vi "Build Octree from triangles.vi"(3 "Triangle array":T4[](array[typedef]), 4 "World Pmin (x, y, z)":sgl[](array[numeric]), 5 "World Pmax (x, y, z)":sgl[](array[numeric]), 6 "Octree resolution (model units)":sgl) -> (0 "Stack error":errorcluster, 1 "Branch levels":i32, 2 "Octree node array":T1[](array[typedef]))   [LabVIEW 2016]
uses:
  Typedefs/Triangle.ctl
  Typedefs/TreeNodeBox.ctl
  Typedefs/Quad.ctl
  Typedefs/Quadplane enum.ctl
  Subroutines/TriVert-in-Box test.vi
  Subroutines/BoxEdges-Tri intersection test.vi
  Subroutines/TriEdges-Box intersection test.vi
  Subroutines/Point-in-Box test (axis-aligned).vi
  Subroutines/Edge-Tri intersection test.vi
  Subroutines/Edge-Quad intersection test.vi
  Subroutines/Point-in-Tri test.vi
  Subroutines/Edge-Plane intersection test.vi
  Subroutines/Point-in-Quad test (axis-aligned).vi
  Subroutines/Dot product.vi
panel:
  out "Octree node stack history":i32(graph)
  # "PN 17/01/2015"
  # "Vertices"
  # "Edges"
  # "Unit normal"
  # "Plane ident."
  # "Vertices"
  # "Edges"
  # "Unit normal"
  # "Plane ident."
  # "Vertices"
  # "Edges"
  # "Unit normal"
  # "Plane ident."
  # "Vertices"
  # "Edges"
  # "Unit normal"
  # "Plane ident."
  # "Vertices"
  # "Edges"
  # "Unit normal"
  # "Plane ident."
  # "Vertices"
  # "Edges"
  # "Unit normal"
  # "Plane ident."
  # "Vertices"
  # "Edges"
  # "Unit normal"
  # "Edge unit normals"
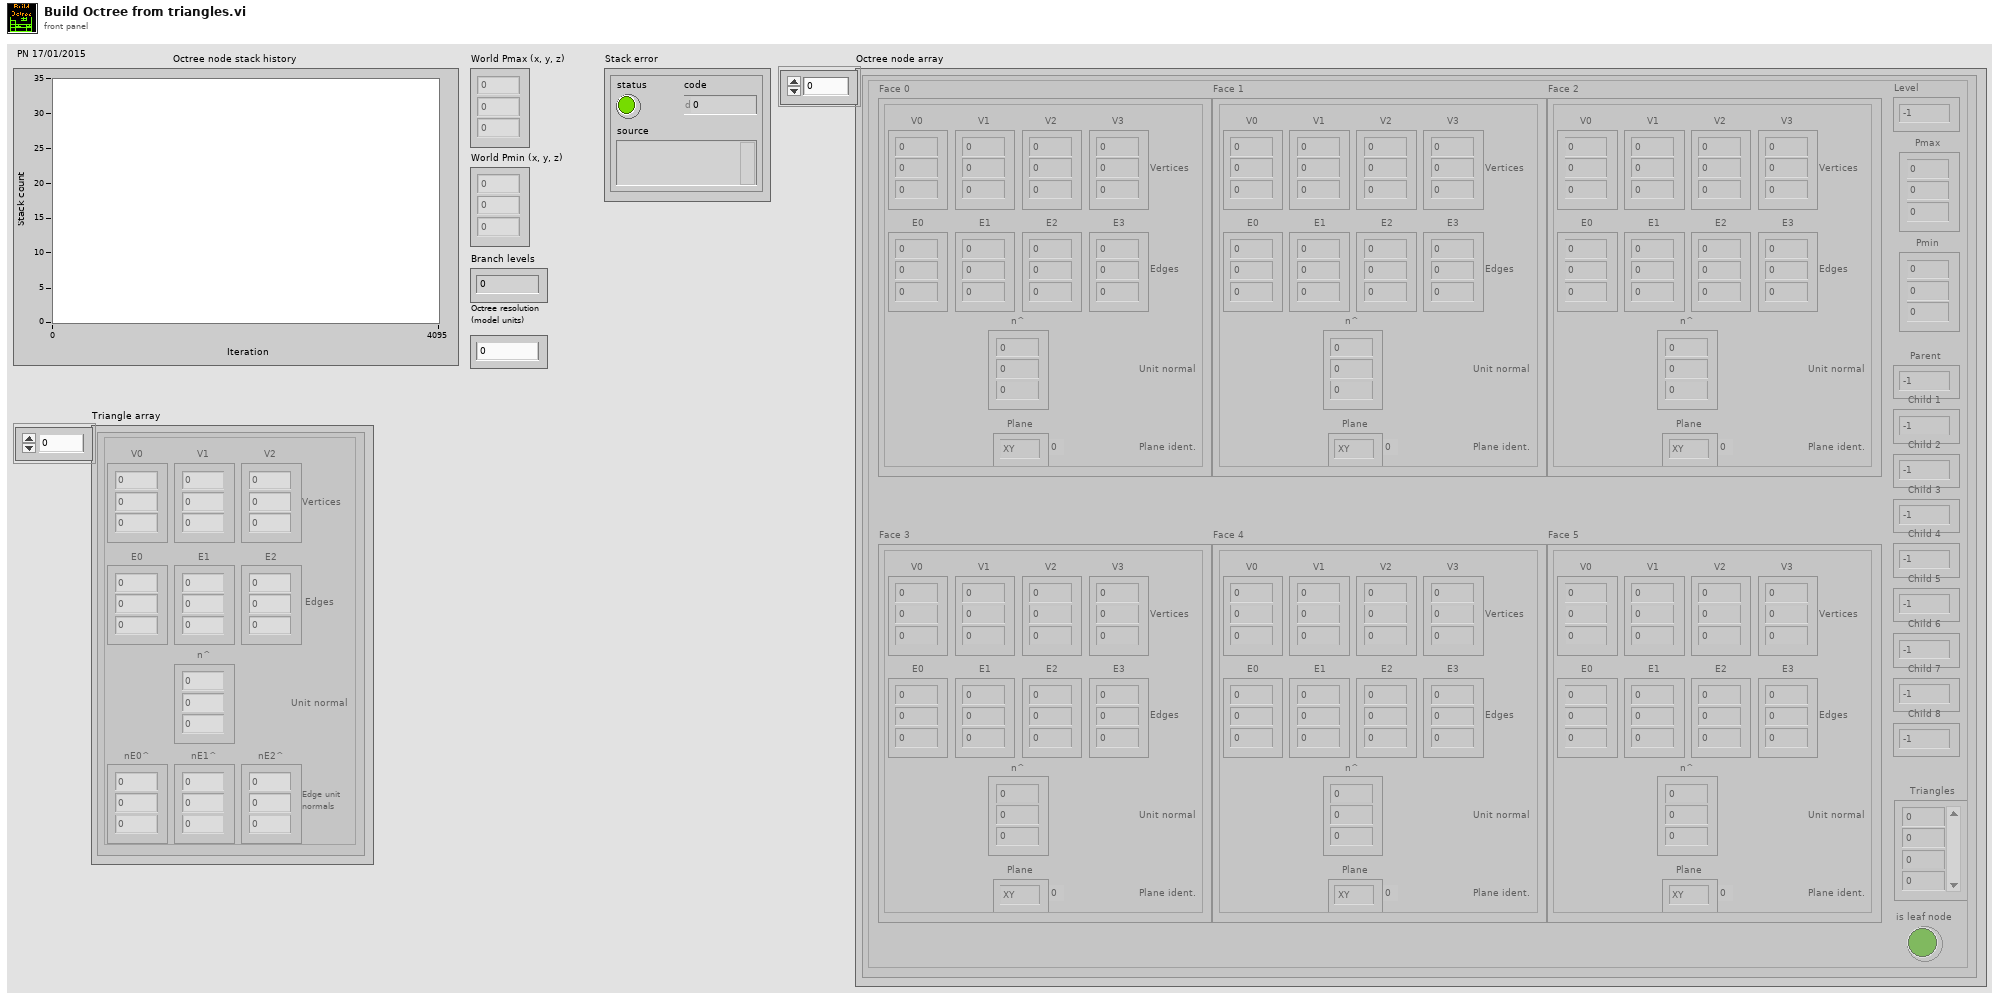
[diagram p1: front panel]
types:
  T1 = typedef "TreeNodeBox.ctl" = cluster{"Face 0":T2, "Face 1":T2, "Face 2":T2, "Face 3":T2, "Face 4":T2, "Face 5":T2, "Level":i32, "Pmax":sgl[], "Pmin":sgl[], "Parent":i32, "Child 1":i32, "Child 2":i32, "Child 3":i32, "Child 4":i32, "Child 5":i32, "Child 6":i32, "Child 7":i32, "Child 8":i32, "Triangles":i32[], "is leaf node":bool}
  T2 = typedef "Quad.ctl" = cluster{"V0":sgl[], "V1":sgl[], "V2":sgl[], "V3":sgl[], "E0":sgl[], "E1":sgl[], "E2":sgl[], "E3":sgl[], "n^":sgl[], "Plane":T3}
  T3 = typedef "Quadplane enum.ctl" = enum8{"XY", "XZ", "YZ", "-XY", "-XZ", "-YZ"}
  T4 = typedef "Triangle.ctl" = cluster{"V0":sgl[], "V1":sgl[], "V2":sgl[], "E0":sgl[], "E1":sgl[], "E2":sgl[], "n^":sgl[], "nE0^":sgl[], "nE1^":sgl[], "nE2^":sgl[]}
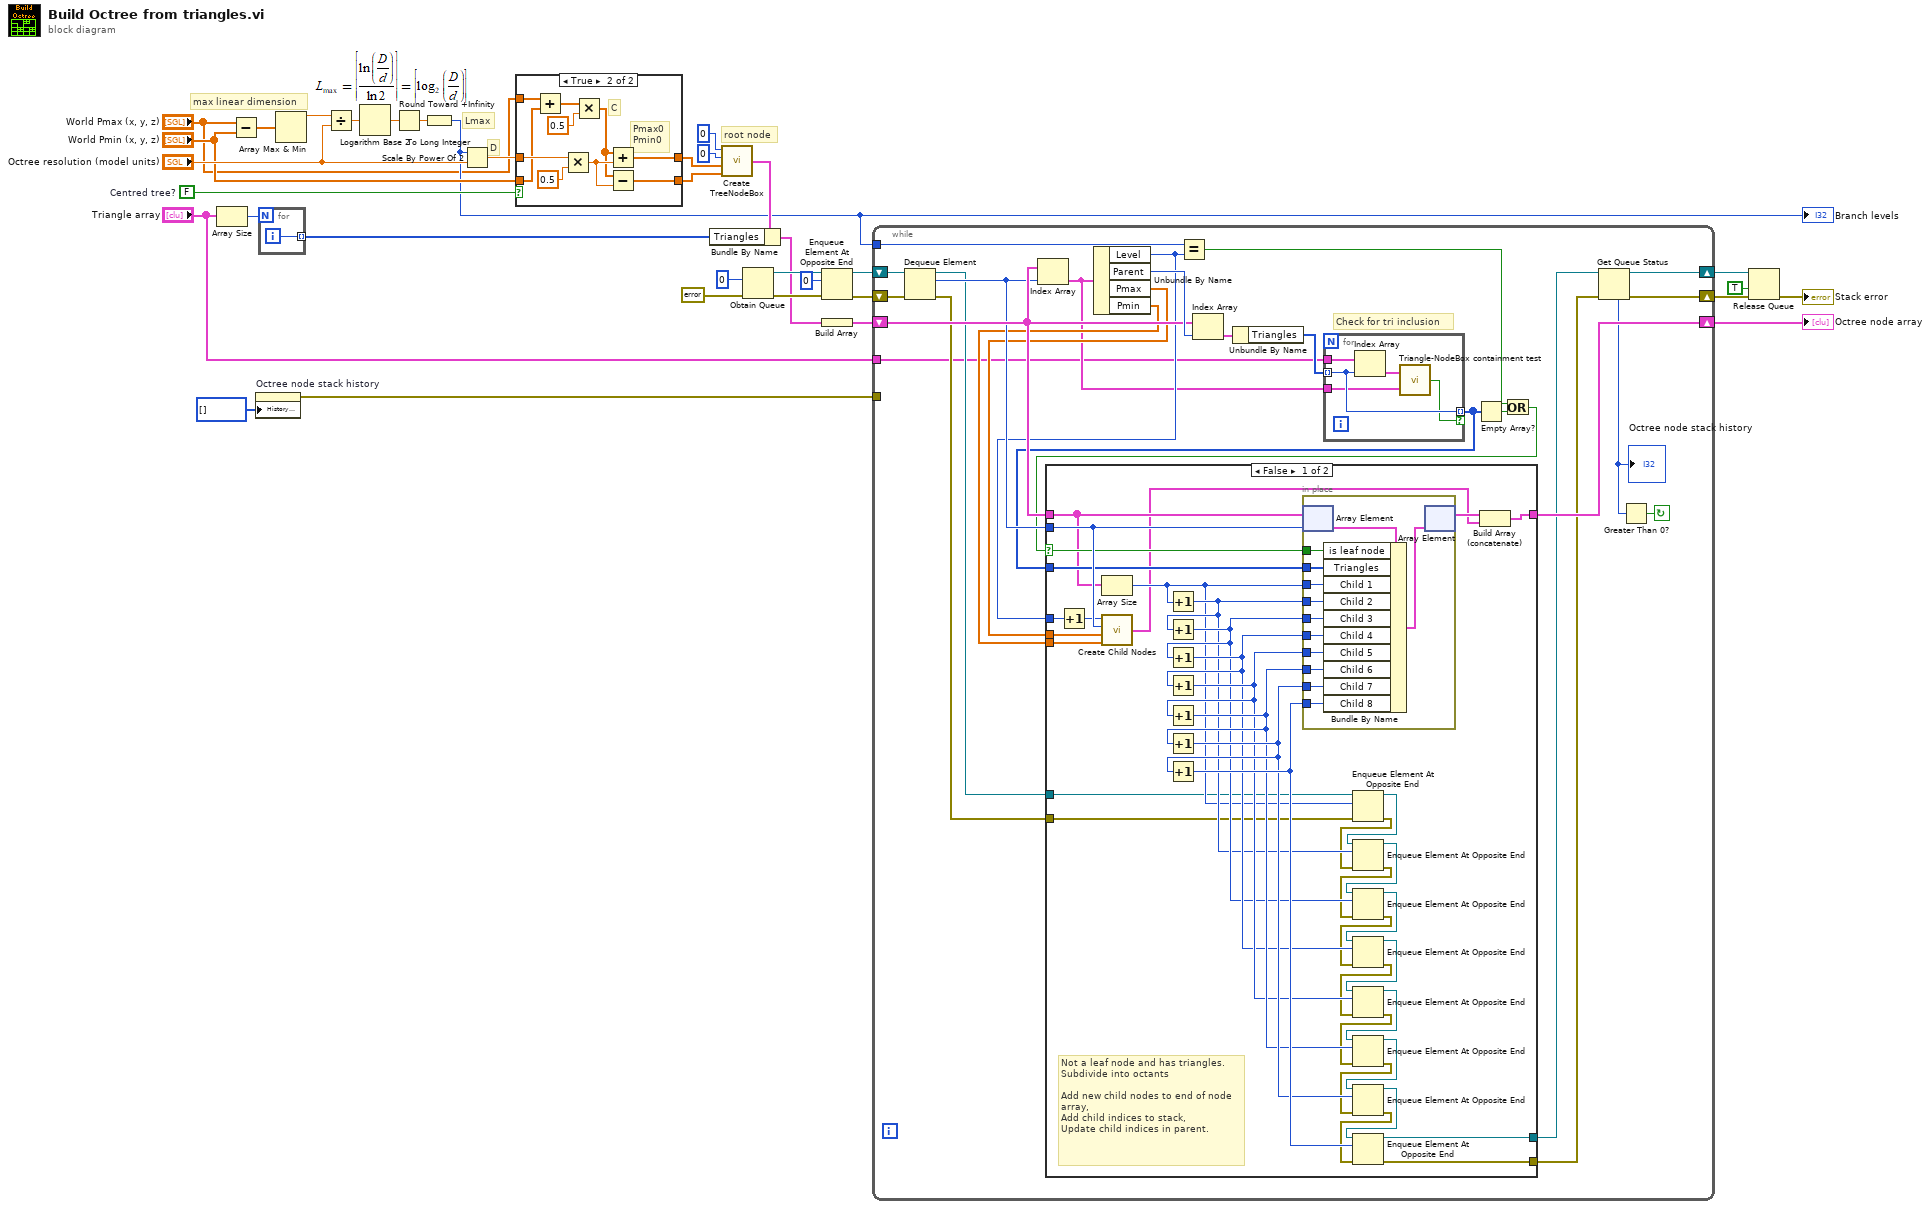
[diagram p0: block diagram]
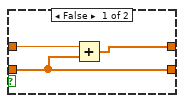
[diagram p2: hidden frame]
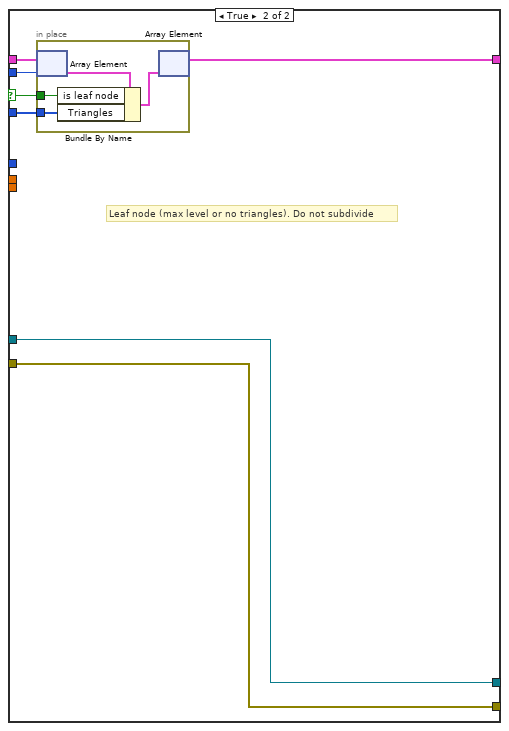
[diagram p3: hidden frame]
diagram:
  w4 = FALSE  # Centred tree?
  # "root node"
  # "D"
  # "Lmax"
  # "max linear dimension"
  n1 = Array Size(array="Triangle array") -> (size(s)=w24:i32)
  n2 = Subtract(x="World Pmax (x, y, z)", y="World Pmin (x, y, z)") -> (x-y=w35:sgl[])
  n3 = property on="Octree node stack history" class="WFChart (strict)"("History Data"=i32[] []) -> (error out=w12:errorcluster)  [unwired: 2 in, 1 out]
  n4 = for {
    N: w24 -> [_]
    tunnel: [w36] -> w23 mode=indexing
    i -> [w36]
  }
  n5 = Array Max & Min(array=w35) -> (max value=w9:sgl)  [unwired: 3 out]
  n6 = Divide(x=w9, y="Octree resolution (model units)") -> (x/y=w34:sgl)
  n7 = Logarithm Base 2(1:w34) -> (0:w33:sgl)
  n8 = Round Toward +Infinity(x=w33) -> (ceil(x): smallest int >= x=w32:sgl)
  n9 = To Long Integer(number=w32) -> (32bit integer=w3:i32)
  "Branch levels" <- w3
  n10 = Scale By Power Of 2(n=w3, x="Octree resolution (model units)") -> (x*2^n=w8:sgl)
  n11 = case shown="True" w4 {
    tunnel: w8 -> [w39 w47]
    tunnel: [w37 w46] -> w5
    tunnel: [w38 w45] -> w6
    tunnel: "World Pmin (x, y, z)" -> [w38 w41]
    tunnel: "World Pmax (x, y, z)" -> [_ w40]
    frame False {
      n12 = Add(x=w39, y=w38) -> (x+y=w37:sgl[])
    }
    frame True {
      # "C"
      # "Pmax0\nPmin0"
      n13 = Add(x=w40, y=w41) -> (x+y=w44:sgl[])
      n14 = Multiply(x=w47, y=sgl 0.5 ("Numeric")) -> (x*y=w48:sgl)
      n15 = Multiply(x=w44, y=sgl 0.5 ("Numeric")) -> (x*y=w42:sgl[])
      n16 = Add(x=w42, y=w48) -> (x+y=w46:sgl[])
      n17 = Subtract(x=w42, y=w48) -> (x-y=w45:sgl[])
    }
  }
  n18 = call "Create TreeNodeBox.vi"("Pmin"=w6, "Pmax"=w5, "Parent"=0, "Level"=0) -> ("Box"=w15:T1)
  n19 = Bundle By Name(cluster=w15, "Triangles"=w23) -> (w22:T1)
  n20 = Obtain Queue(element data type=0, error in (no error)=errorcluster {"status"=FALSE, "code"=0, "source"=""}) -> (queue out=w30:refnum<queue>, error out=w29:errorcluster)  [unwired: 3 in, 1 out]
  n21 = Enqueue Element At Opposite End(queue=w30, element=0, error in (no error)=w29) -> (queue out=w28:refnum<queue>, error out=w27:errorcluster)  [unwired: 1 in, 1 out]
  n22 = Build Array(w22) -> (w21:T1[])
  n23 = while {
    shift-right: [w57] -> w26
    shift-left: w28 -> [w75]
    shift-right: [w72] -> w25
    shift-left: w27 -> [w74]
    shift-right: [w60] -> w18
    shift-left: w21 -> [w65]
    tunnel: w3 -> [w68]
    tunnel: w12 -> [_]
    tunnel: "Triangle array" -> [w50]
    stop <- w73 continue-if-true
    # "Check for tri inclusion"
    n24 = Dequeue Element(queue=w75, error in (no error)=w74) -> (queue out=w56:refnum<queue>, element=w64:i32, error out=w55:errorcluster)  [unwired: 1 in, 1 out]
    n25 = Index Array(array=w65, index=w64) -> (element=w51:T1)
    n26 = Unbundle By Name(w51) -> ("Level"=w62:i32, "Parent"=w70:i32, "Pmax"=w58:sgl[], "Pmin"=w59:sgl[])
    n27 = Equal?(x=w68, y=w62) -> (x = y?=w66:bool)
    n28 = Index Array(array=w65, index=w70) -> (element=w69:T1)
    n29 = Unbundle By Name(w69) -> ("Triangles"=w71:i32[])
    n30 = for {
      tunnel: w71 -> [w139] mode=indexing
      tunnel: [w139] -> w63 mode=indexing if=w138
      tunnel: w51 -> [w137]
      tunnel: w50 -> [w136]
      n31 = Index Array(array=w136, index=w139) -> (element=w140:T4)
      n32 = call "Triangle-NodeBox containment test.vi"("NodeBox"=w137, "Triangle"=w140) -> ("Triangle is in NodeBox"=w138:bool)
    }
    n33 = Empty Array?(array=w63) -> (empty?=w67:bool)
    n34 = Or(x=w66, y=w67) -> (x .or. y?=w61:bool)
    n35 = case shown="False" w61 {
      selector: w61 -> [w108 w128]
      tunnel: w65 -> [w105 w131]
      tunnel: w64 -> [w112 w130]
      tunnel: w63 -> [w111 w129]
      tunnel: w62 -> [w110 _]
      tunnel: [w104 w127] -> w60
      tunnel: w59 -> [w107 _]
      tunnel: w58 -> [w106 _]
      tunnel: w56 -> [w92 w126]
      tunnel: [w79 w126] -> w54
      tunnel: [w78 w125] -> w53
      tunnel: w55 -> [w77 w125]
      frame False {
        # "Not a leaf node and has triangles.\nSubdivide into octants\n\nAdd new child nodes to end of node array,\nAdd child indices to stack,\nUpdate child indices in parent."
        n36 = Increment(x=w110) -> (x+1=w109:i32)
        n37 = Array Size(array=w105) -> (size(s)=w95:i32)
        n38 = call "Create Child Nodes.vi"("Pmin (parent)"=w107, "Pmax (parent)"=w106, "Parent"=w112, "Level (parent+1)"=w109) -> ("8 Child nodes array"=w76:T1[])
        n39 = Increment(x=w95) -> (x+1=w96:i32)
        n40 = Increment(x=w96) -> (x+1=w97:i32)
        n41 = Increment(x=w97) -> (x+1=w98:i32)
        n42 = Increment(x=w98) -> (x+1=w99:i32)
        n43 = Increment(x=w99) -> (x+1=w100:i32)
        n44 = Increment(x=w100) -> (x+1=w101:i32)
        n45 = Increment(x=w101) -> (x+1=w102:i32)
        n46 = in-place {
          in-place-border: w108 -> [w122]
          in-place-border: w111 -> [w121]
          in-place-border: w95 -> [w120]
          in-place-border: w96 -> [w119]
          in-place-border: w97 -> [w118]
          in-place-border: w98 -> [w117]
          in-place-border: w99 -> [w116]
          in-place-border: w100 -> [w115]
          in-place-border: w101 -> [w114]
          in-place-border: w102 -> [w113]
          n47 = in-place-array #1(w105, w112) -> (w124:T1)
          n48 = Bundle By Name(cluster=w124, "is leaf node"=w122, "Triangles"=w121, "Child 1"=w120, "Child 2"=w119, "Child 3"=w118, "Child 4"=w117, "Child 5"=w116, "Child 6"=w115, "Child 7"=w114, "Child 8"=w113) -> (w123:T1)
          n49 = in-place-array #1(w123) -> (w103:T1[])  [unwired: 1 out]
        }
        n50 = Enqueue Element At Opposite End(queue=w92, element=w95, error in (no error)=w77) -> (queue out=w93:refnum<queue>, error out=w94:errorcluster)  [unwired: 1 in, 1 out]
        n51 = Enqueue Element At Opposite End(queue=w93, element=w96, error in (no error)=w94) -> (queue out=w91:refnum<queue>, error out=w90:errorcluster)  [unwired: 1 in, 1 out]
        n52 = Enqueue Element At Opposite End(queue=w91, element=w97, error in (no error)=w90) -> (queue out=w88:refnum<queue>, error out=w89:errorcluster)  [unwired: 1 in, 1 out]
        n53 = Enqueue Element At Opposite End(queue=w88, element=w98, error in (no error)=w89) -> (queue out=w86:refnum<queue>, error out=w87:errorcluster)  [unwired: 1 in, 1 out]
        n54 = Enqueue Element At Opposite End(queue=w86, element=w99, error in (no error)=w87) -> (queue out=w84:refnum<queue>, error out=w85:errorcluster)  [unwired: 1 in, 1 out]
        n55 = Enqueue Element At Opposite End(queue=w84, element=w100, error in (no error)=w85) -> (queue out=w82:refnum<queue>, error out=w83:errorcluster)  [unwired: 1 in, 1 out]
        n56 = Enqueue Element At Opposite End(queue=w82, element=w101, error in (no error)=w83) -> (queue out=w80:refnum<queue>, error out=w81:errorcluster)  [unwired: 1 in, 1 out]
        n57 = Enqueue Element At Opposite End(queue=w80, element=w102, error in (no error)=w81) -> (queue out=w79:refnum<queue>, error out=w78:errorcluster)  [unwired: 1 in, 1 out]
        n58 = Build Array (concatenate)(w103, w76) -> (w104:T1[])
      }
      frame True {
        # "Leaf node (max level or no triangles). Do not subdivide"
        n59 = in-place {
          in-place-border: w128 -> [w133]
          in-place-border: w129 -> [w132]
          n60 = in-place-array #2(w131, w130) -> (w135:T1)
          n61 = Bundle By Name(cluster=w135, "is leaf node"=w133, "Triangles"=w132) -> (w134:T1)
          n62 = in-place-array #2(w134) -> (w127:T1[])  [unwired: 1 out]
        }
      }
    }
    n63 = Get Queue Status(queue=w54, error in (no error)=w53) -> (queue out=w57:refnum<queue>, error out=w72:errorcluster, # elements in queue=w52:i32)  [unwired: 1 in, 5 out]
    "Octree node stack history" <- w52
    n64 = Greater Than 0?(x=w52) -> (x > 0?=w73:bool)
  }
  "Octree node array" <- w18
  n65 = Release Queue(queue=w26, force destroy? (F)=TRUE, error in (no error)=w25) -> (error out=→"Stack error":errorcluster)  [unwired: 2 out]
